vi "Application Mode Change.vi"(8 "error in (no error)":errorcluster, 10 "Mode":T1, 11 "Main Window in":refnum<class "Main Window.lvclass">) -> (0 "error out":errorcluster, 3 "Main Window out":refnum<class "Main Window.lvclass">)   [LabVIEW 2018, in "Main Window.lvlib" / "Main Window.lvclass"]
uses:
  Main Window.lvclass
  Application/Mode.ctl
  Main Window.lvclass/Main Window.ctl
  Application/Application.lvlib
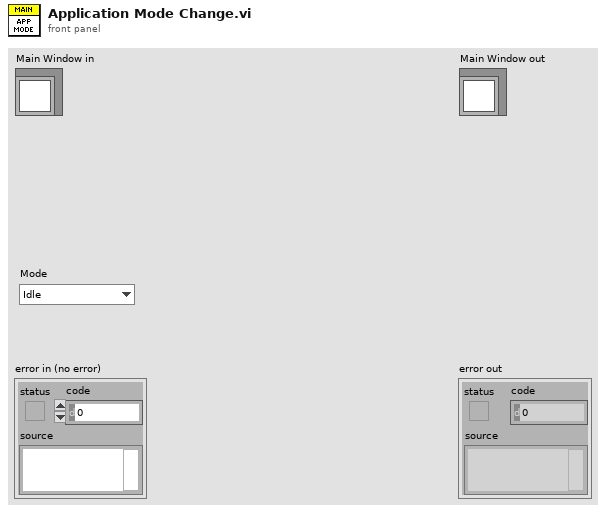
[diagram p1: front panel]
types:
  T1 = typedef "Application.lvlib/Mode.ctl" = enum16{"Idle", "Live", "Stream", "Autofocus", "Z-Stack"}
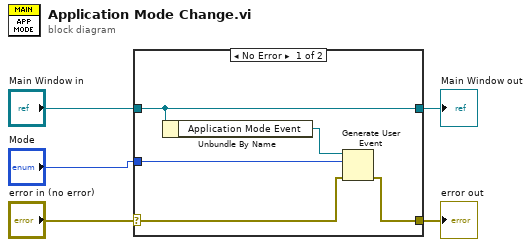
[diagram p0: block diagram]
diagram:
  n1 = case shown="No Error" "error in (no error)" {
    selector: "error in (no error)" -> [w9 w12]
    tunnel: [w8 w12] -> w4
    tunnel: [w7 w11] -> w2
    tunnel: "Main Window in" -> [w7 w11]
    tunnel: "Mode" -> [w10 _]
    frame No Error {
      n2 = Unbundle By Name(w7) -> ("Application Mode Event"=w6:refnum<user-event>)
      n3 = Generate User Event(user event=w6, event data cluster=w10, error in=w9) -> (error out=w8:errorcluster)  [unwired: 1 in, 1 out]
    }
    frame Error {
    }
  }
  "error out" <- w4
  "Main Window out" <- w2
